vi "Get all LabVIEW INI keys.vi"(8 "error in (no error)":errorcluster) -> (0 "error out":errorcluster, 3 "INI Keys":T1[](array[typedef]))   [LabVIEW 2015, in "RT Management.lvlib"]
doc: "Gets all INI keys from a given INI file located in the data folder and bundles them up with the Section, Key Name, and Key Value."
uses:
  RT Management.lvlib
  controls/INI key.ctl
  <vilib>/Utility/config.llb/Read Key (String).vi
  <vilib>/Utility/config.llb/NI_LVConfig.lvlib
panel:
  in  "configuration file path":path
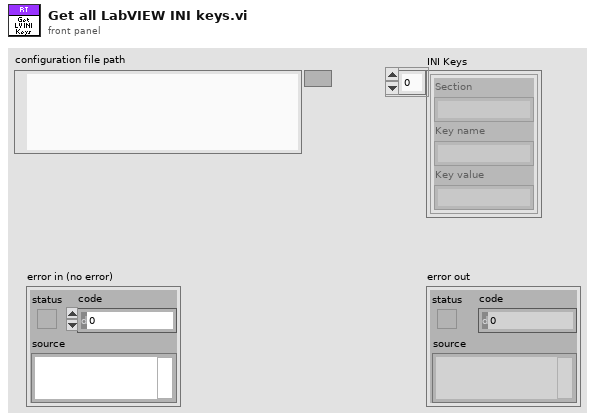
[diagram p1: front panel]
types:
  T1 = typedef "RT Management.lvlib/INI key.ctl" = cluster{"Section":string, "Key name":string, "Key value":string}
  T2 = typedef "NI_LVConfig.lvlib/Config Data RefNum.ctl" = refnum<k1>
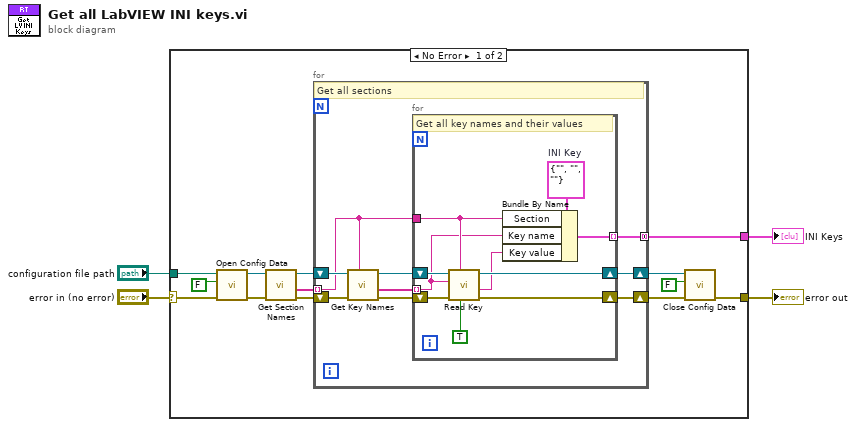
[diagram p0: block diagram]
diagram:
  n1 = case shown="No Error" "error in (no error)" {
    selector: "error in (no error)" -> [w7 w37]
    tunnel: [w8 w37] -> w4
    tunnel: [w6 _] -> w2
    tunnel: "configuration file path" -> [w5 _]
    frame No Error {
      n2 = call <vilib>:"Open Config Data.vi"("error in (no error)"=w7, "create file if necessary (T)"=FALSE, "configuration file path"=w5) -> ("error out"=w16:errorcluster, "refnum"=w15:T2)  [unwired: 6 in, 1 out]
      n3 = call <vilib>:"Get Section Names.vi"("error in (no error)"=w16, "refnum"=w15) -> ("error out"=w13:errorcluster, "section names"=w12:string[], "refnum out"=w14:T2)  [unwired: 7 in]
      n4 = for {
        tunnel: w12 -> [w21] mode=indexing
        tunnel: [w18] -> w6 mode=concatenating
        shift-right: [w20] -> w10
        shift-left: w14 -> [w25]
        shift-right: [w19] -> w11
        shift-left: w13 -> [w26]
        # "Get all sections"
        n5 = call <vilib>:"Get Key Names.vi"("section"=w21, "error in (no error)"=w26, "refnum"=w25) -> ("error out"=w24:errorcluster, "key names"=w22:string[], "refnum out"=w23:T2)  [unwired: 5 in, 1 out]
        n6 = for {
          tunnel: w22 -> [w33] mode=indexing
          tunnel: w21 -> [w34]
          tunnel: [w28] -> w18 mode=indexing
          shift-right: [w31] -> w20
          shift-left: w23 -> [w35]
          shift-right: [w32] -> w19
          shift-left: w24 -> [w36]
          w29 = T1 {"Section"="", "Key name"="", "Key value"=""}  # INI Key
          # "Get all key names and their values"
          n7 = call-poly <vilib>:"Read Key.vi"("read raw string? (F)"=TRUE, "section"=w34, "error in (no error)"=w36, "key"=w33, "refnum"=w35) -> ("error out"=w32:errorcluster, "value"=w30:string, "refnum out"=w31:T2)  [unwired: 3 in, 1 out]
          n8 = Bundle By Name(cluster=w29, "Section"=w34, "Key name"=w33, "Key value"=w30) -> (w28:T1)
        }
      }
      n9 = call <vilib>:"Close Config Data.vi"("error in (no error)"=w11, "write file if changed (T)"=FALSE, "refnum"=w10) -> ("error out"=w8:errorcluster)  [unwired: 7 in, 1 out]
    }
    frame Error {
    }
  }
  "error out" <- w4
  "INI Keys" <- w2
